vi "New Session SetUp.vi"(8 "error in (no error)":errorcluster, 10 "Stop Refnum":refnum<vi>, 11 "Abstract Sensor in":refnum<class "Abstract Sensor.lvclass">) -> (0 "error out":errorcluster, 3 "Abstract Sensor out":refnum<class "Abstract Sensor.lvclass">)   [LabVIEW 2014, in "Abstract Sensor.lvlib" / "Abstract Sensor.lvclass"]
uses:
  Abstract Sensor.lvclass
  Generic Instrument/Generic Instrument.lvclass
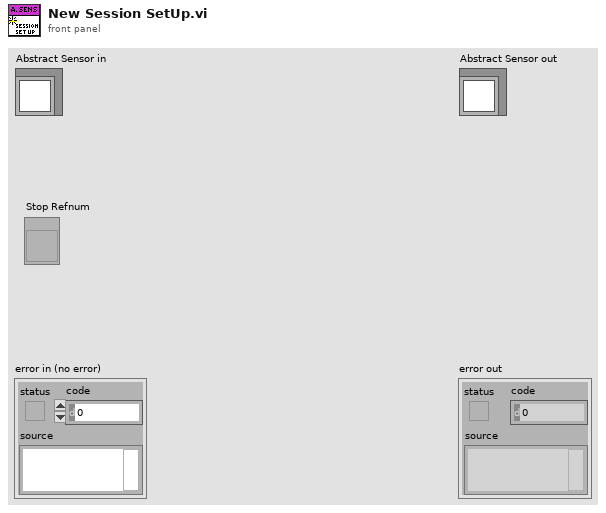
[diagram p1: front panel]
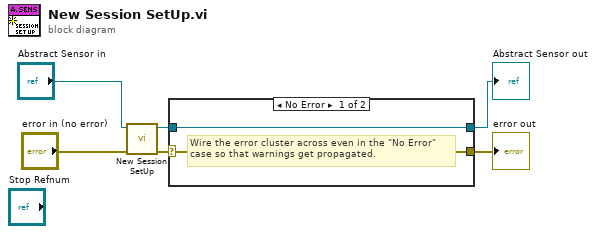
[diagram p0: block diagram]
diagram:
  n1 = call-parent "New Session SetUp.vi"("error in (no error)"="error in (no error)", "Generic Instrument in"="Abstract Sensor in") -> ("error out"=w1:errorcluster, "Generic Instrument out"=w3:refnum<class "Abstract Sensor.lvclass">)  [unwired: 8 in]
  n2 = case shown="No Error" w1 {
    selector: w1 -> [w7 w10]
    tunnel: [w7 w10] -> w6
    tunnel: [w8 w9] -> w5
    tunnel: w3 -> [w8 w9]
    frame No Error {
      # "Wire the error cluster across even in the \"No Error\"\ncase so that warnings get propagated."
    }
    frame Error {
    }
  }
  "error out" <- w6
  "Abstract Sensor out" <- w5
